vi "Global Variable.vi"() -> ()   [LabVIEW 2021]
panel:
  in  "Values":dbl[](array[numeric])
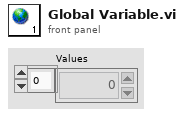
[diagram p1: front panel]
diagram:
